vi "Oculus Rift Guidance().vi"() -> (3 "Guidance Library.lvlib:Oculus Rift Guidance.lvclass":refnum<class "Oculus Rift Guidance.lvclass">)   [LabVIEW 2014, in "Guidance Library.lvlib" / "Oculus Rift Guidance.lvclass"]
uses:
  Oculus Rift Guidance.lvclass
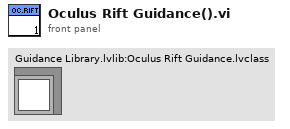
[diagram p1: front panel]
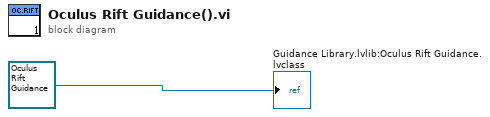
[diagram p0: block diagram]
diagram:
  "Guidance Library.lvlib:Oculus Rift Guidance.lvclass" <- refnum<class "Oculus Rift Guidance.lvclass"> refnum ("Guidance Library.lvlib:Oculus Rift Guidance.lvclass")
